vi "Binomial Moments.vi"(9 "p":dbl=0.02, 10 "n":i32=100) -> (0 "error":i32, 2 "variance":dbl=1.96, 3 "mean":dbl=2.0)   [LabVIEW 2020, in "NI_Gmath.lvlib"]
doc: "Returns the expected mean and variance of the random variate X, where X describes the selected distribution type. You must manually select the polymorphic instance to use."
uses:
  <vilib>/gmath/NI_Gmath.lvlib
  <vilib>/gmath/statdist.llb/st_error_code.ctl
panel:
  # "Binomial Moments"
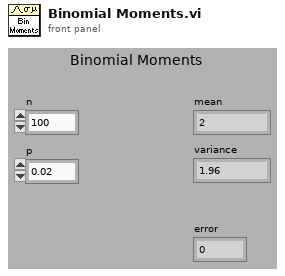
[diagram p1: front panel]
types:
  T1 = typedef "NI_Gmath.lvlib/st_error_code.ctl" = i32
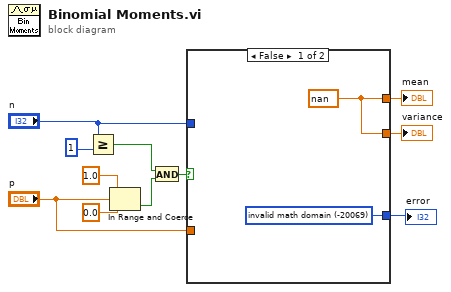
[diagram p0: block diagram]
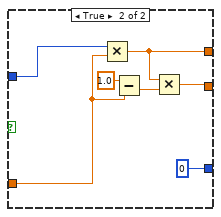
[diagram p2: hidden frame]
diagram:
  n1 = Greater Or Equal?(x="n", y=1) -> (x >= y?=w6:bool)
  n2 = In Range and Coerce(upper limit=1.0, x="p", lower limit=0.0) -> (In Range?=w5:bool)  [unwired: 1 out]
  n3 = And(x=w6, y=w5) -> (x .and. y?=w1:bool)
  n4 = case shown="False" w1 {
    tunnel: [w13 w15] -> w11
    tunnel: [w13 w14] -> w10
    tunnel: [w12 0 ("error")] -> w2
    tunnel: "n" -> [_ w19]
    tunnel: "p" -> [_ w17]
    frame False {
      w12 = T1 -20069 items=["invalid math domain"=-20069, "Fourier interpolation size m >= n"=-20070, "empty array"=-20003] ("stat interp error code")
      w13 = nan
    }
    frame True {
      n5 = Multiply(x=w19, y=w17) -> (x*y=w15:dbl)
      n6 = Subtract(x=1.0, y=w17) -> (x-y=w16:dbl)
      n7 = Multiply(x=w15, y=w16) -> (x*y=w14:dbl)
    }
  }
  "error" <- w2
  "mean" <- w11
  "variance" <- w10
